vi "niDTS BT INSTR TX UTILChar Select.vi"(7 "Character Select":enum16{"DF1", "DF2"}(ring)) -> (8 "ModulationCharacteristicSelction":enum16{"DF1", "DF2"}(ring))   [LabVIEW 2015, in "niDTS BT.lvlib" / "niDTS BT INSTR TX.lvclass"]
uses:
  niDTS BT INSTR TX.lvclass
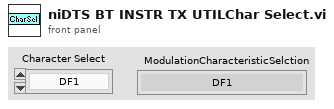
[diagram p1: front panel]
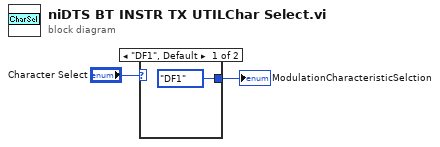
[diagram p0: block diagram]
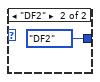
[diagram p2: hidden frame]
diagram:
  n1 = case shown="\"DF1\", Default" "Character Select" {
    tunnel: [enum16{"DF1", "DF2"}."DF1" ("ModulationCharacteristicSelction") enum16{"DF1", "DF2"}."DF2" ("ModulationCharacteristicSelction")] -> w1
    frame "DF1", Default {
    }
    frame "DF2" {
    }
  }
  "ModulationCharacteristicSelction" <- w1
